vi "Test Modes.vi"(8 "error in (no error)":errorcluster, 11 "Instrument.Lockin in":refnum<class "Instrument.Lockin.lvclass">) -> (0 "error out":errorcluster, 3 "Instrument.Lockin out":refnum<class "Instrument.Lockin.lvclass">)   [LabVIEW 2016]
uses:
  src/Instrument.Lockin/Instrument.Lockin.lvclass
  src/Instrument.Lockin/Typedefs/AO_Channel-Numeric.ctl
  <vilib>/addons/_JKI Toolkits/Caraya/classes/Assert/Assert Not Error.vi
  <vilib>/addons/_JKI Toolkits/Caraya/classes/Assert/Assert Equal Value_Variant.vi
  <vilib>/addons/_JKI Toolkits/Caraya/classes/Assert/Assert Not Equal Value and Type_Variant.vi
  <vilib>/addons/_JKI Toolkits/Caraya/classes/Test/Test.lvclass
  <vilib>/addons/_JKI Toolkits/Caraya/classes/Assert/Assert.lvclass
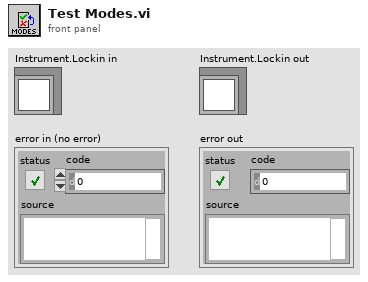
[diagram p1: front panel]
types:
  T1 = typedef "Instrument.Lockin.lvclass/AO_Channel-Numeric.ctl" = i32
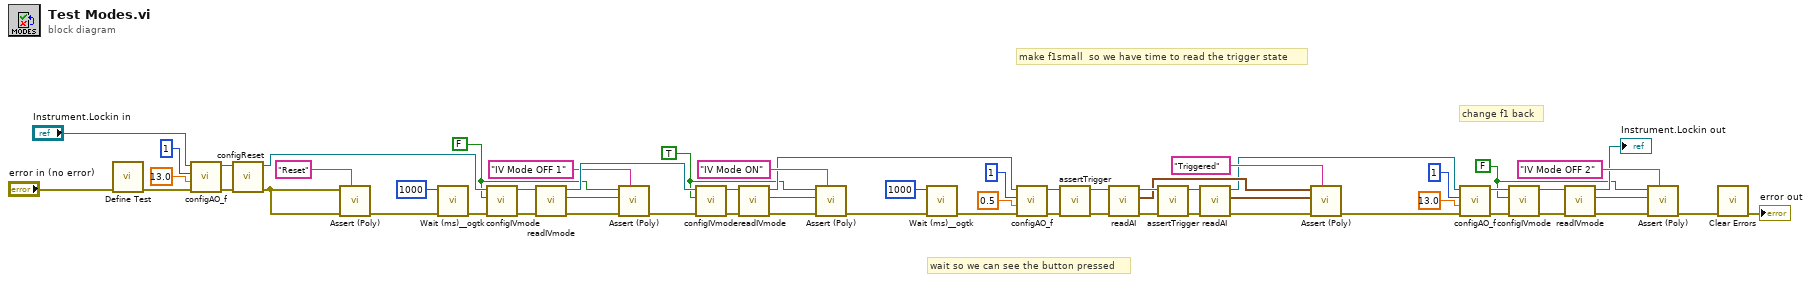
[diagram p0: block diagram]
diagram:
  w20 = FALSE ("IV mode")
  w25 = FALSE ("IV mode")
  w22 = TRUE ("IV mode")
  # "change f1 back"
  # "make f1small  so we have time to read the trigger state"
  # "wait so we can see the button pressed"
  n1 = call <vilib>:"Define Test.vi"("error in (no error)"="error in (no error)") -> ("error out"=w3:errorcluster)  [unwired: 10 in]
  n2 = call "configAO_f.vi"("error in (no error)"=w3, "Frequency (Hz)"=13.0, "AO Channel"=T1 1, "Instrument.Lockin in"="Instrument.Lockin in") -> ("error out"=w4:errorcluster, "Instrument.Lockin out"=w2:refnum<class "Instrument.Lockin.lvclass">)  [unwired: 6 in]
  n3 = call "configReset.vi"("error in (no error)"=w4, "Instrument.Lockin in"=w2) -> ("error out"=w50:errorcluster, "Instrument.Lockin out"=w32:refnum<class "Instrument.Lockin.lvclass">)  [unwired: 8 in]
  n4 = call-poly <vilib>:"Assert (Poly).vi"("Label"="Reset", "error in (no error)"=w50, "Not Error?"=w50) -> ("error out"=w18:errorcluster)  [unwired: 8 in]
  n5 = call <userlib>:"Wait (ms)__ogtk.vi"("error in (no error)"=w18, "milliseconds to wait"=u32 1000) -> ("error out"=w17:errorcluster)  [unwired: 8 in, 1 out]
  n6 = call "configIVmode.vi"("error in (no error)"=w17, "IV mode"=w20, "Instrument.Lockin in"=w32) -> ("error out"=w30:errorcluster, "Instrument.Lockin out"=w31:refnum<class "Instrument.Lockin.lvclass">)  [unwired: 7 in]
  n7 = call "readIVmode.vi"("error in (no error)"=w30, "Instrument.Lockin in"=w31) -> ("error out"=w28:errorcluster, "IV mode"=w21:bool, "Instrument.Lockin out"=w29:refnum<class "Instrument.Lockin.lvclass">)  [unwired: 7 in]
  n8 = call-poly <vilib>:"Assert (Poly).vi"("Label"="IV Mode OFF 1", "error in (no error)"=w28, "Y"=w21, "X"=w20) -> ("error out"=w27:errorcluster)  [unwired: 7 in]
  n9 = call "configIVmode.vi"("error in (no error)"=w27, "IV mode"=w22, "Instrument.Lockin in"=w29) -> ("error out"=w59:errorcluster, "Instrument.Lockin out"=w58:refnum<class "Instrument.Lockin.lvclass">)  [unwired: 7 in]
  n10 = call "readIVmode.vi"("error in (no error)"=w59, "Instrument.Lockin in"=w58) -> ("error out"=w55:errorcluster, "IV mode"=w23:bool, "Instrument.Lockin out"=w42:refnum<class "Instrument.Lockin.lvclass">)  [unwired: 7 in]
  n11 = call-poly <vilib>:"Assert (Poly).vi"("Label"="IV Mode ON", "error in (no error)"=w55, "Y"=w23, "X"=w22) -> ("error out"=w45:errorcluster)  [unwired: 7 in]
  n12 = call <userlib>:"Wait (ms)__ogtk.vi"("error in (no error)"=w45, "milliseconds to wait"=u32 1000) -> ("error out"=w43:errorcluster)  [unwired: 8 in, 1 out]
  n13 = call "configAO_f.vi"("error in (no error)"=w43, "Frequency (Hz)"=0.5, "AO Channel"=T1 1, "Instrument.Lockin in"=w42) -> ("error out"=w39:errorcluster, "Instrument.Lockin out"=w38:refnum<class "Instrument.Lockin.lvclass">)  [unwired: 6 in]
  n14 = call "assertTrigger.vi"("error in (no error)"=w39, "Instrument.Lockin in"=w38) -> ("error out"=w16:errorcluster, "Instrument.Lockin out"=w15:refnum<class "Instrument.Lockin.lvclass">)  [unwired: 8 in]
  n15 = call "readAI.vi"("error in (no error)"=w16, "Instrument.Lockin in"=w15) -> ("error out"=w14:errorcluster, "AI Waveform"=w9:waveform(dbl)[], "Instrument.Lockin out"=w13:refnum<class "Instrument.Lockin.lvclass">)  [unwired: 7 in]
  n16 = call "assertTrigger.vi"("error in (no error)"=w14, "Instrument.Lockin in"=w13) -> ("error out"=w12:errorcluster, "Instrument.Lockin out"=w11:refnum<class "Instrument.Lockin.lvclass">)  [unwired: 8 in]
  n17 = call "readAI.vi"("error in (no error)"=w12, "Instrument.Lockin in"=w11) -> ("error out"=w8:errorcluster, "AI Waveform"=w10:waveform(dbl)[], "Instrument.Lockin out"=w7:refnum<class "Instrument.Lockin.lvclass">)  [unwired: 7 in]
  n18 = call-poly <vilib>:"Assert (Poly).vi"("Label"="Triggered", "error in (no error)"=w8, "Y"=w10, "X"=w9) -> ("error out"=w35:errorcluster)  [unwired: 7 in]
  n19 = call "configAO_f.vi"("error in (no error)"=w35, "Frequency (Hz)"=13.0, "AO Channel"=T1 1, "Instrument.Lockin in"=w7) -> ("error out"=w34:errorcluster, "Instrument.Lockin out"=w33:refnum<class "Instrument.Lockin.lvclass">)  [unwired: 6 in]
  n20 = call "configIVmode.vi"("error in (no error)"=w34, "IV mode"=w25, "Instrument.Lockin in"=w33) -> ("error out"=w56:errorcluster, "Instrument.Lockin out"=w57:refnum<class "Instrument.Lockin.lvclass">)  [unwired: 7 in]
  n21 = call "readIVmode.vi"("error in (no error)"=w56, "Instrument.Lockin in"=w57) -> ("error out"=w52:errorcluster, "IV mode"=w24:bool, "Instrument.Lockin out"=→"Instrument.Lockin out":refnum<class "Instrument.Lockin.lvclass">)  [unwired: 7 in]
  n22 = call-poly <vilib>:"Assert (Poly).vi"("Label"="IV Mode OFF 2", "error in (no error)"=w52, "Y"=w24, "X"=w25) -> ("error out"=w48:errorcluster)  [unwired: 7 in]
  n23 = call <vilib>:"Clear Errors.vi"("error in (no error)"=w48) -> ("error out"=→"error out":errorcluster)  [unwired: 5 in, 1 out]
